vi "XDOUT.VI"(2 "?":u32 format="%.0x", 3 "PortNum":i32(ring)=1 items=["AUXPORT", "FIRSTPORTA", "FIRSTPORTB", "FIRSTPORTCL", "FIRSTPORTCH", "SECONDPORTA", "SECONDPORTB", "SECONDPORTCL", "SECONDPORTCH", "THIRDPORTA", "THIRDPORTB", "THIRDPORTCL", "THIRDPORTCH", "FOURTHPORTA", "FOURTHPORTB", "FOURTHPORTCL", "FOURTHPORTCH", "FIFTHPORTA", "FIFTHPORTB", "FIFTHPORTCL", "FIFTHPORTCH", "SIXTHPORTA", "SIXTHPORTB", "SIXTHPORTCL", "SIXTHPORTCH", "SEVENTHPORTA", "SEVENTHPORTB", "SEVENTHPORTCL", "SEVENTHPORTCH", "EIGTHPORTA", "EIGHTHPORTB", "EIGHTHPORTCL", "EIGHTHPORTCH"], 4 "BoardNum":u32) -> ()   [LabVIEW 2013]
panel:
  out "DOut ErrMsg":string
  out "DConfigPort ErrMsg":string
  # "Demo for the DOut.VI and DCfgPort.VI corresponding to the Universal Library functions  cbDOut() and cbDConfigPort().\n\nConfigures the digital port and outputs the value to the port."
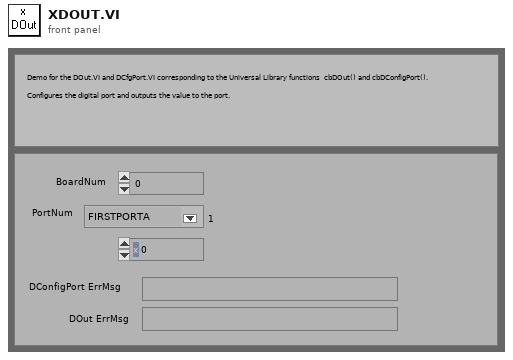
[diagram p1: front panel]
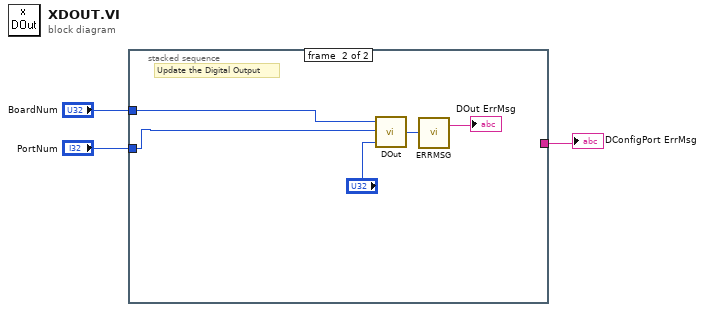
[diagram p0: block diagram]
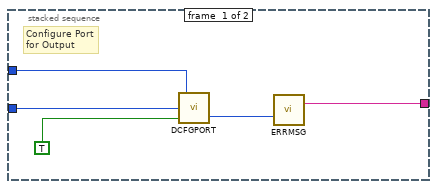
[diagram p2: hidden frame]
diagram:
  n1 = stacked-sequence {
    tunnel: [w8 _] -> w3
    tunnel: "BoardNum" -> [w5 w13]
    tunnel: "PortNum" -> [w4 w12]
    frame #0 {
      # "Configure Port \nfor Output"
      n2 = call "DCFGPORT.VI"("Direction"=TRUE, "PortNum"=w4, "BoardNum"=w5) -> ("ErrCode"=w7:i32)  [unwired: 1 out]
      n3 = call "ERRMSG.VI"("ErrCode"=w7) -> ("ErrMsg"=w8:string)  [unwired: 1 out]
    }
    frame #1 {
      # "Update the Digital Output"
      n4 = call "DOut.VI"("DataValue"="?", "PortNum"=w12, "BoardNum"=w13) -> ("ErrCode"=w10:i32)
      n5 = call "ERRMSG.VI"("ErrCode"=w10) -> ("ErrMsg"=→"DOut ErrMsg":string)  [unwired: 1 out]
    }
  }
  "DConfigPort ErrMsg" <- w3
